vi "GetInfo.vi"(11 "File selected":T2) -> (2 "remove?":bool)   [LabVIEW 2022 SP3]
uses:
  Curtin1_Label.ctl
panel:
  in  "Instruments":u16(ring) items=["ME45 01 H.AvR", "ME45 02 H.AvR", "ME45 03 H.AvR"]
  in  "Play":bool
  in  "View Raw Data":bool
  in  "Open":bool
  out "Block":bool
  in  "Done 2":bool
  out "Instrument--Test":string
  in  "Recalc":bool
  in  "Overwrite":bool
  in  "Settings":T1={"Name of test"="", "Date"=timestamp(0 s since 1904-01-01), "Location"="", "Default Template"="", "Soundcard"="", "resolution"=32, "Sampling rate"=48000, "Ch1 Gain "=25.0, "Ch2 Gain"=10.0, "Sample time (s)"=0.3, "Pre-trigger (s)"=0.01, "Hammer Threshold"=10.0, "Positions"=12, "Taps/Position"=5, "Set Names"="", "Freq resolution"=10.0, "Hammer cutoff"=0.0, "Mic cutoff"=0.0, "Double bounce "=0.0, "Hammer Cal"=10.0, "dB Offset"=0.0, "Accel Cal"=10.0, "Vibrometer Cal"=0.0, "Mic Cal"=0.0, "Output"=2, "Voltage Cal"=0.01, "Vibrometer Port"="ASRL27::INSTR", "Range"=4, "High Pass"=2, "Bandwidth"=4, "X Range"=[{"Minimum"=200.0, "Maximum"=10000.0, "Increment"=10.0, "Minor Increment"=100.0, "Start"=200.0}, {"Minimum"=0.0, "Maximum"=0.05, "Increment"=0.025, "Minor Increment"=0.0025, "Start"=0.0}, {"Minimum"=0.0, "Maximum"=0.3, "Increment"=0.1, "Minor Increment"=0.01, "Start"=0.0}, {"Minimum"=200.0, "Maximum"=10000.0, "Increment"=10.0, "Minor Increment"=100.0, "Start"=1000.0}], "Y Range"=[{"Minimum"=-25.0, "Maximum"=0.0, "Increment"=5.0, "Minor Increment"=1.0, "Start"=-25.0}, {"Minimum"=-0.01, "Maximum"=0.1, "Increment"=0.02, "Minor Increment"=0.005, "Start"=0.0}, {"Minimum"=-0.1, "Maximum"=0.1, "Increment"=0.05, "Minor Increment"=0.01, "Start"=-0.1}, {"Minimum"=-35.0, "Maximum"=5.0, "Increment"=2.0, "Minor Increment"=0.5, "Start"=-34.0}], "dB Spread"=0.0, "Trigger"=0, "Ch_1"=25, "Ch_2"=25, "flip?"=FALSE, "60Hz"=FALSE, "Time offset"=0.0, "Piezo Cal"=0.0, "Default Notes"="", "Tom"=FALSE} {"Ch_2" min=1 step=1; "Ch_1" min=1 max=100 step=1; "Trigger" items=["Hammer (force)", "Self-tap"]; "Bandwidth" items=["1 kHz", "5 kHz", "10 kHz", "25 kHz", "50 kHz", "100 kHz"]; "High Pass" items=["Off", "13 Hz", "104 Hz"]; "Range" items=["10 mm/s", "20 mm/s", "50 mm/s", "100 mm/s", "200 mm/s", "500 mm/s", "1 m/s", "2 m/s"]; "Output" items=["Acclerometer", "Displacement", "Microphone", "Vibrometer"]; "Voltage Cal" format="%#_13g"; "Ch2 Gain" format="%#_13g"; "Ch1 Gain" format="%#_13g"; "Hammer Cal" min=0.0; "Double bounce" min=0.0; "Mic cutoff" min=0.0 format="%#_4g"; "Hammer cutoff" min=0.0 format="%#_4g"; "Freq resolution" min=0.0; "Pre-trigger (s)" format="%#_13g"; "Date" format="%<%H:%M\n%d/%m/%y>T"; "resolution" items=["16 bit"=16, "24 bit"=24, "32 bit"=32]; "Sampling rate" items=["22050 samp/s"=22050, "44100 samp/s"=44100, "48000 samp/s"=48000]}
  in  "Save as a Template":bool
  in  "Save":bool
  in  "Done":bool
  out "Tags":string
  in  "Notes":string
  out "File name":string
  # "mV/Pa"
  # "mV/m/s2"
  # "mV/mm/s"
  # "V/N"
  # "sec"
  # "sec"
  # "mV/N"
  # "Hz"
  # "a.u."
  # "dB"
  # "a.u."
  # "dB"
  # "sec"
  # "sec"
  # "sec"
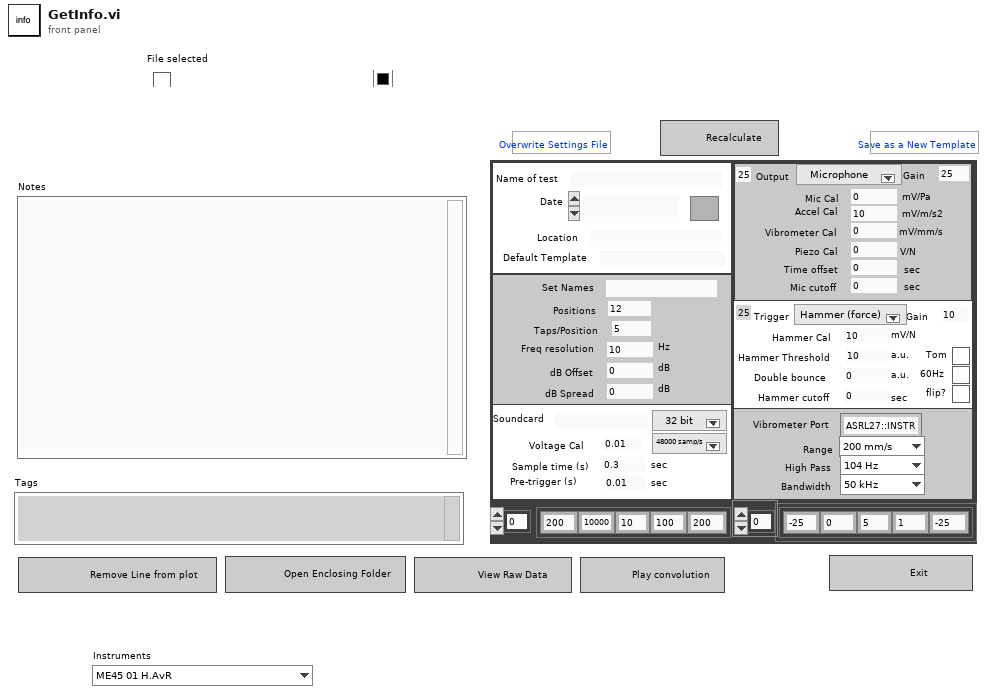
[diagram p1: front panel]
types:
  T1 = cluster{"Name of test":string, "Date":timestamp, "Location":string, "Default Template":string, "Soundcard":string, "resolution":u16, "Sampling rate":u16, "Ch1 Gain ":dbl, "Ch2 Gain":dbl, "Sample time (s)":dbl, "Pre-trigger (s)":dbl, "Hammer Threshold":dbl, "Positions":i16, "Taps/Position":i16, "Set Names":string, "Freq resolution":dbl, "Hammer cutoff":dbl, "Mic cutoff":dbl, "Double bounce ":dbl, "Hammer Cal":dbl, "dB Offset":dbl, "Accel Cal":dbl, "Vibrometer Cal":dbl, "Mic Cal":dbl, "Output":u16, "Voltage Cal":dbl, "Vibrometer Port":string, "Range":u16, "High Pass":u16, "Bandwidth":u16, "X Range":cluster{"Minimum":dbl, "Maximum":dbl, "Increment":dbl, "Minor Increment":dbl, "Start":dbl}[], "Y Range":cluster{"Minimum":dbl, "Maximum":dbl, "Increment":dbl, "Minor Increment":dbl, "Start":dbl}[], "dB Spread":dbl, "Trigger":u16, "Ch_1":u8, "Ch_2":u8, "flip?":bool, "60Hz":bool, "Time offset":dbl, "Piezo Cal":dbl, "Default Notes":string, "Tom":bool}
  T2 = typedef "Curtin1_Label.ctl" = cluster{"Show?":bool, "Name":string, "Color":u32, "Path":path, "Show Notes":bool}
  T3 = enum8{"Enabled", "Disabled", "Disabled and Grayed Out"}
  T4 = cluster{"Name of test":string, "Date":timestamp, "Location":string, "Template":string, "Soundcard":string, "resolution":u16, "Sampling rate":u16, "Ch1 Gain ":dbl, "Ch2 Gain":dbl, "Sample time (s)":dbl, "Pre-trigger (s)":dbl, "Hammer Threshold":dbl, "Positions":i16, "Taps/Position":i16, "Set Names":string, "Freq resolution":dbl, "Hammer cutoff":dbl, "Mic cutoff":dbl, "Double bounce ":dbl, "Hammer Cal":dbl, "dB Offset":dbl, "Accel Cal":dbl, "Vibrometer Cal":dbl, "Mic Cal":dbl, "Output":u16, "Voltage Cal":dbl, "Vibrometer Port":string, "Range":u16, "High Pass":u16, "Bandwidth":u16, "X Range":cluster{"Minimum":dbl, "Maximum":dbl, "Increment":dbl, "Minor Increment":dbl, "Start":dbl}[], "Y Range":cluster{"Minimum":dbl, "Maximum":dbl, "Increment":dbl, "Minor Increment":dbl, "Start":dbl}[], "dB Spread":dbl, "Trigger":u16, "Ch_1":u8, "Ch_2":u8, "flip?":bool, "60Hz":bool, "Time offset":dbl, "Piezo Cal":dbl, "Default Notes":string, "Tom":bool}
  T5 = enum32{"Invalid", "Default", "Floating", "Floating/Auto-Hide", "Modal"}
  T6 = typedef "PreferencesControl.ctl" = cluster{"Name of test":string, "Date":timestamp, "Location":string, "Template":string, "Soundcard":string, "resolution":u16, "Sampling rate":u16, "Ch1 Gain ":dbl, "Ch2 Gain":dbl, "Sample time (s)":dbl, "Pre-trigger (s)":dbl, "Hammer Threshold":dbl, "Positions":i16, "Taps/Position":i16, "Set Names":string, "Freq resolution":dbl, "Hammer cutoff":dbl, "Mic cutoff":dbl, "Double bounce ":dbl, "Hammer Cal":dbl, "dB Offset":dbl, "Accel Cal":dbl, "Vibrometer Cal":dbl, "Mic Cal":dbl, "Output":u16, "Voltage Cal":dbl, "Vibrometer Port":refnum<visa-resource-name>, "Range":u16, "High Pass":u16, "Bandwidth":u16, "X Range":cluster{"Minimum":dbl, "Maximum":dbl, "Increment":dbl, "Minor Increment":dbl, "Start":dbl}[], "Y Range":cluster{"Minimum":dbl, "Maximum":dbl, "Increment":dbl, "Minor Increment":dbl, "Start":dbl}[], "dB Spread":dbl, "Trigger":u16, "Ch_1":u8, "Ch_2":u8, "flip?":bool, "60Hz":bool, "Time offset":dbl, "Piezo Cal":dbl, "Default Notes":string, "Tom":bool}
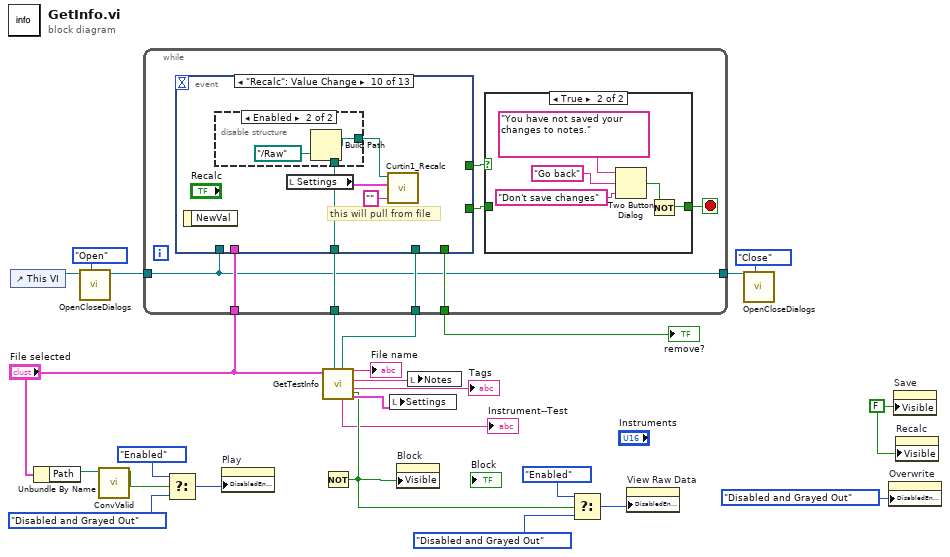
[diagram p0: block diagram]
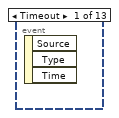
[diagram p3: hidden frame]
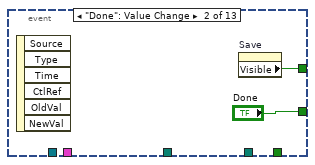
[diagram p4: hidden frame]
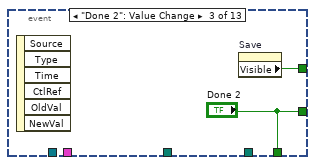
[diagram p5: hidden frame]
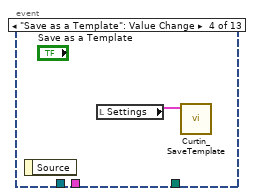
[diagram p6: hidden frame]
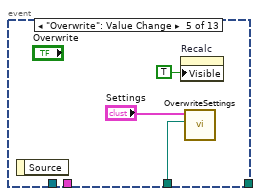
[diagram p7: hidden frame]
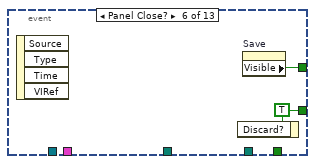
[diagram p8: hidden frame]
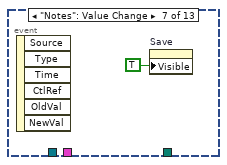
[diagram p9: hidden frame]
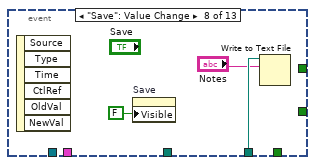
[diagram p10: hidden frame]
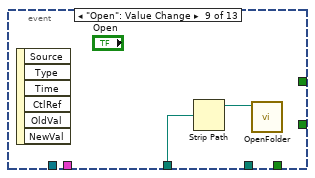
[diagram p11: hidden frame]
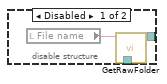
[diagram p12: hidden frame]
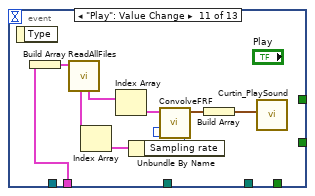
[diagram p13: hidden frame]
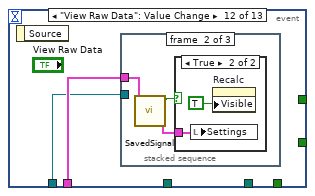
[diagram p14: hidden frame]
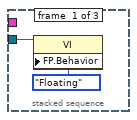
[diagram p15: hidden frame]
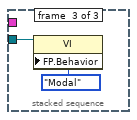
[diagram p17: hidden frame]
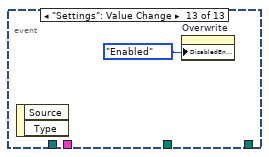
[diagram p18: hidden frame]
diagram:
  w26 = FALSE ("Visible")
  n1 = control-ref of="This VI"() -> (w16:refnum<vi>)
  n2 = Unbundle By Name("File selected") -> ("Path"=w3:path)
  n3 = call "OpenCloseDialogs.vi"("Task"=enum16{"Open", "Close"}."Open", "VI in"=w16) -> ("VI out"=w13:refnum<vi>)  [unwired: 8 in, 1 out]
  n4 = call "ConvValid.vi"("Path"=w3) -> ("Valid"=w2:bool)  [unwired: 10 in]
  n5 = Select(t=T3."Enabled" ("Disabled"), s=w2, f=T3."Disabled and Grayed Out" ("Disabled")) -> (s? t:f=w6:T3)
  n6 = property on="Play" class="Bool"("DisabledEnum"=w6) -> ()  [unwired: 2 in, 2 out]
  n7 = call "GetTestInfo.vi"("File selected"="File selected") -> ("Settings"=w21:T4, "Tags"=→"Tags":string, "Notes"=w23:string, "File name"=→"File name":string, "Instrument--Test"=→"Instrument--Test":string, "Notes Path"=w19:path, "Visible?"=w10:bool, "Settings Path"=w20:path)  [unwired: 3 in]
  n8 = while {
    tunnel: w19 -> [w34]
    tunnel: w20 -> [w30]
    tunnel: [w29] -> w18
    tunnel: [w27] -> w14
    tunnel: w13 -> [w27]
    tunnel: "File selected" -> [w28]
    stop <- w31 stop-if-true
    n9 = event shown="[9] \"Recalc\": Value Change" {
      selector: _ -> [_ _ _ _ _ _ _ _ _ _ _ _ _]
      dyn-events: _ -> [_ _ _ _ _ _ _ _ _ _ _ _ _]
      timeout: _ -> [_ _ _ _ _ _ _ _ _ _ _ _ _]
      tunnel: w34 -> [_ _ _ _ _ _ _ w54 _ _ _ _ _]
      tunnel: [_ w42 w44 _ _ w50 _ _ _ _ _ _ _] -> w33
      tunnel: [_ "Done" "Done 2" _ _ w49 _ _ _ _ _ _ _] -> w32
      tunnel: w30 -> [_ _ _ _ w47 _ _ _ w56 w58 _ _ _]
      tunnel: [_ _ "Done 2" _ _ _ _ _ _ _ _ _ _] -> w29
      tunnel: w28 -> [_ _ _ _ _ _ _ _ _ _ w67 w76 _]
      tunnel: w27 -> [_ _ _ _ _ _ _ _ _ _ _ w75 _]
      event Timeout {
        n10 = event-data() -> ()  [unwired: 1 in, 3 out]
      }
      event "Done": Value Change {
        n11 = event-data() -> ()  [unwired: 1 in, 6 out]
        n12 = property on="Save" class="Bool"() -> ("Visible"=w42:bool)  [unwired: 2 in, 2 out]
      }
      event "Done 2": Value Change {
        n13 = event-data() -> ()  [unwired: 1 in, 6 out]
        n14 = property on="Save" class="Bool"() -> ("Visible"=w44:bool)  [unwired: 2 in, 2 out]
      }
      event "Save as a Template": Value Change {
        n15 = event-data() -> ()  [unwired: 1 in, 1 out]
        n16 = local read "Settings"() -> (w45:T1)
        n17 = call "Curtin_SaveTemplate.vi"("Settings in"=w45) -> ()  [unwired: 8 in, 3 out]
      }
      event "Overwrite": Value Change {
        n18 = event-data() -> ()  [unwired: 1 in, 1 out]
        n19 = property on="Recalc" class="Bool"("Visible"=TRUE) -> ()  [unwired: 2 in, 2 out]
        n20 = call "OverwriteSettings.vi"("Settings path"=w47, "Settings"="Settings") -> ()  [unwired: 9 in, 1 out]
      }
      event Panel Close? {
        w49 = TRUE ("Done")
        n21 = event-data() -> ()  [unwired: 1 in, 4 out]
        n22 = event-data("Discard?"=w49) -> ()  [unwired: 1 in, 1 out]
        n23 = property on="Save" class="Bool"() -> ("Visible"=w50:bool)  [unwired: 2 in, 2 out]
      }
      event "Notes": Value Change {
        n24 = event-data() -> ()  [unwired: 1 in, 6 out]
        n25 = property on="Save" class="Bool"("Visible"=TRUE) -> ()  [unwired: 2 in, 2 out]
      }
      event "Save": Value Change {
        n26 = event-data() -> ()  [unwired: 1 in, 6 out]
        n27 = property on="Save" class="Bool"("Visible"=FALSE) -> ()  [unwired: 2 in, 2 out]
        n28 = Write to Text File(file (use dialog)=w54, text="Notes") -> ()  [unwired: 2 in, 3 out]
      }
      event "Open": Value Change {
        n29 = event-data() -> ()  [unwired: 1 in, 6 out]
        n30 = Strip Path(path=w56) -> (stripped path=w55:path)  [unwired: 1 out]
        n31 = call "OpenFolder.vi"("LabVIEW Data Path"=w55) -> ()  [unwired: 11 in]
      }
      event "Recalc": Value Change {
        # "this will pull from file"
        n32 = event-data() -> ()  [unwired: 1 in, 1 out]
        n33 = disable-structure shown="Enabled" {
          disable-tunnel: [w61 w63] -> w59
          disable-tunnel: w58 -> [_ w64]
          frame Disabled {
            n34 = local read "File name"() -> (w62:string)
            n35 = call "GetRawFolder.vi"("File name"=w62) -> ("Path to Raw data"=w61:path)  [unwired: 10 in]
          }
          frame Enabled {
            n36 = Build Path(base path=w64, name or relative path=path "../Raw") -> (appended path=w63:path)
          }
        }
        n37 = local read "Settings"() -> (w60:T1)
        n38 = call "Curtin1_Recalc.vi"("Instrument:Test Name"="", "Settings"=w60, "Path To Raw Folder"=w59) -> ()  [unwired: 9 in]
      }
      event "Play": Value Change {
        n39 = event-data() -> ()  [unwired: 1 in, 1 out]
        n40 = Build Array(w67) -> (w66:T2[])
        n41 = call "ReadAllFiles.vi"("Files"=w66) -> ("data"=w68:cluster{"t0":dbl, "df":dbl, "Y":cdb[]}[], "Settings"=w70:T6[])  [unwired: 5 in, 4 out]
        n42 = Index Array(array=w70) -> (element=w71:T6)  [unwired: 1 in]
        n43 = Index Array(array=w68) -> (element=w69:cluster{"t0":dbl, "df":dbl, "Y":cdb[]})  [unwired: 1 in]
        n44 = Unbundle By Name(w71) -> ("Sampling rate"=w72:u16)
        n45 = call "ConvolveFRF.vi"("Sampling rate"=w72, "Complex FRF"=w69) -> ("Convolution"=w73:waveform(dbl))  [unwired: 6 in, 3 out]
        n46 = Build Array(w73) -> (w74:waveform(dbl)[])
        n47 = call "Curtin_PlaySound.vi"("all waveforms"=w74) -> ()  [unwired: 10 in, 1 out]
      }
      event "View Raw Data": Value Change {
        n48 = event-data() -> ()  [unwired: 1 in, 1 out]
        n49 = stacked-sequence {
          tunnel: w76 -> [_ w81 _]
          tunnel: w75 -> [w77 _ w84]
          frame #0 {
            n50 = property class="VI"(reference=w77, "FP.Behavior"=T5."Floating" ("Front Panel Window:Behavior")) -> ()  [unwired: 1 in, 2 out]
          }
          frame #1 {
            n51 = call "SavedSignal.vi"("File selected"=w81) -> ("Settings out"=w79:T6, "update?"=w80:bool)  [unwired: 9 in]
            n52 = case shown="True" w80 {
              tunnel: w79 -> [_ w82]
              frame False {
              }
              frame True {
                n53 = local write "Settings"(w82) -> ()
                n54 = property on="Recalc" class="Bool"("Visible"=TRUE) -> ()  [unwired: 2 in, 2 out]
              }
            }
          }
          frame #2 {
            n55 = property class="VI"(reference=w84, "FP.Behavior"=T5."Modal" ("Front Panel Window:Behavior")) -> ()  [unwired: 1 in, 2 out]
          }
        }
      }
      event "Settings": Value Change {
        n56 = event-data() -> ()  [unwired: 1 in, 2 out]
        n57 = property on="Overwrite" class="Bool"("DisabledEnum"=T3."Enabled" ("Disabled")) -> ()  [unwired: 2 in, 2 out]
      }
    }
    n58 = case shown="True" w33 {
      tunnel: [w35 w36] -> w31
      tunnel: w32 -> [w35 _]
      frame False {
      }
      frame True {
        n59 = Two Button Dialog(message="You have not saved your changes to notes.", 1:"Don't save changes" ("F button name (\"Cancel\")"), 2:"Go back" ("T button name (\"OK\")")) -> (T button?=w37:bool)
        n60 = Not(x=w37) -> (.not. x?=w36:bool)
      }
    }
  }
  "remove?" <- w18
  n61 = Not(x=w10) -> (.not. x?=w12:bool)
  n62 = local write "Settings"(w21) -> ()
  n63 = property on="Block" class="Bool (strict)"("Visible"=w12) -> ()  [unwired: 2 in, 2 out]
  n64 = local write "Notes"(w23) -> ()
  n65 = Select(t=T3."Enabled" ("Disabled"), s=w10, f=T3."Disabled and Grayed Out" ("Disabled")) -> (s? t:f=w8:T3)
  n66 = property on="View Raw Data" class="Bool"("DisabledEnum"=w8) -> ()  [unwired: 2 in, 2 out]
  n67 = call "OpenCloseDialogs.vi"("Task"=enum16{"Open", "Close"}."Close", "VI in"=w14) -> ()  [unwired: 8 in, 2 out]
  n68 = property on="Overwrite" class="Bool"("DisabledEnum"=T3."Disabled and Grayed Out" ("Disabled")) -> ()  [unwired: 2 in, 2 out]
  n69 = property on="Save" class="Bool"("Visible"=w26) -> ()  [unwired: 2 in, 2 out]
  n70 = property on="Recalc" class="Bool"("Visible"=w26) -> ()  [unwired: 2 in, 2 out]
